vi "find first and last common samples.vi"(6 "use_sync_lock":i32, 7 "last_sample":cluster{}, 9 "first_sample":cluster{}, 10 "nFiles":i32, 11 "files_in":string) -> (1 "first_sample out":cluster{}, 2 "function return":i32, 3 "files_in out":string, 5 "last_sample out":cluster{})   [LabVIEW 2019, in "apdm.lvlib"]
doc: "APDM_EXPORT int apdm_find_first_and_last_common_samples(char **files_in, const int nFiles, uint64_t *first_sample, uint64_t *last_sample, const int use_sync_lock);"
uses:
  apdm.lvlib
  Lee Lab/CP FES Walking 2018/Code/Working/LabVIEW/apdm.dll
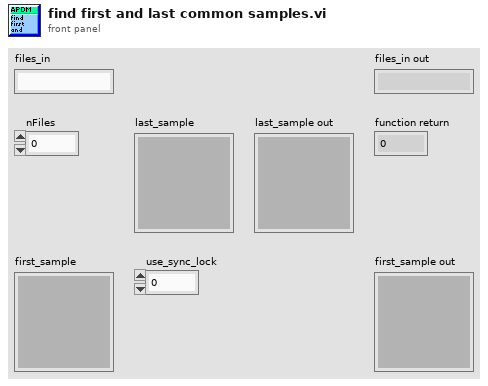
[diagram p1: front panel]
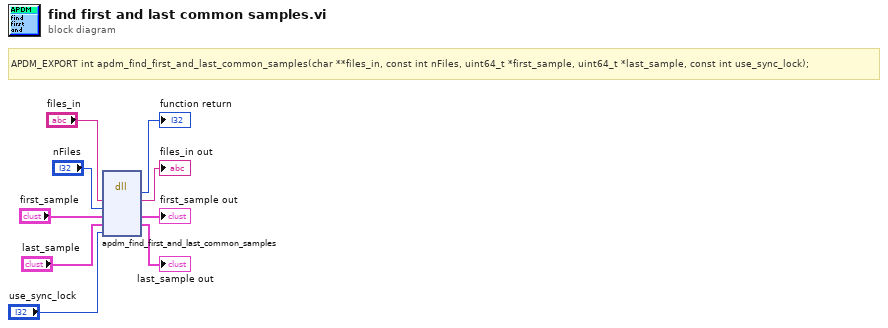
[diagram p0: block diagram]
diagram:
  # "APDM_EXPORT int apdm_find_first_and_last_common_samples(char **files_in, const int nFiles, uint64_t *first_sample, uint64_t *last_sample, const int use_sync_lock);"
  n1 = dll-call lib="C:/Users/jfalesi/Dropbox/Lee Lab/CP FES Walking 2018/Code/Working/LabVIEW/apdm.*" fn="apdm_find_first_and_last_common_samples"("files_in"="files_in", "nFiles"="nFiles", "first_sample"="first_sample", "last_sample"="last_sample", "use_sync_lock"="use_sync_lock") -> (→"function return":i32, "files_in"=→"files_in out":string, "first_sample"=→"first_sample out":cluster{}, "last_sample"=→"last_sample out":cluster{})  [unwired: 5 in, 2 out]
